vi "setUp.vi"(8 "error in (no error)":errorcluster, 11 "reference in":refnum<class "Read Value Tests.lvclass">) -> (0 "error out":errorcluster, 3 "reference out":refnum<class "Read Value Tests.lvclass">)   [LabVIEW 2020, in "Memory Manager Tests.lvlib" / "Read Value Tests.lvclass"]
doc: "setUp runs prior to the test method during test execution. Use this method to initialize any object data required by your tests."
uses:
  Read Value Tests.lvclass
  C:/Program Files (x86)/National Instruments/LabVIEW 2020/vi.lib/addons/_JKI Toolkits/VI Tester/TestCase.llb/TestCase.lvclass
  Read Value Tests.lvclass/Read Value Tests.ctl
  Source/Classes/Pointer/Write 1D U8.vi
  <vilib>/addons/_JKI Toolkits/VI Tester/TestCase.llb/TestCase.lvclass
  Source/Classes/Pointer/Pointer.lvclass
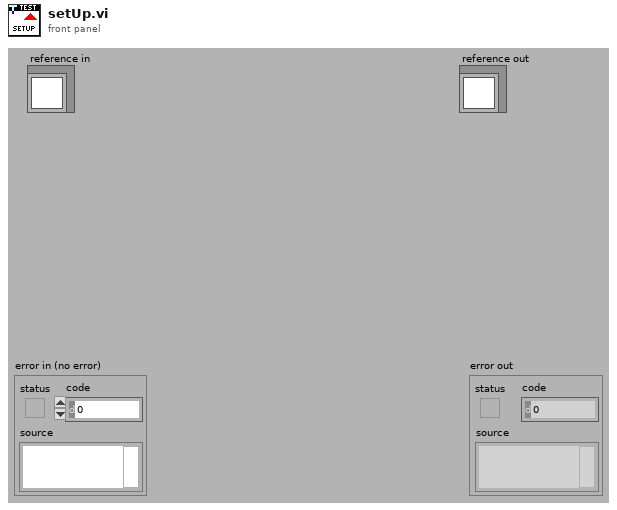
[diagram p1: front panel]
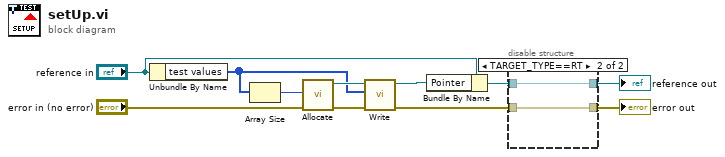
[diagram p0: block diagram]
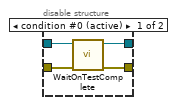
[diagram p2: hidden frame]
diagram:
  n1 = Unbundle By Name("reference in") -> ("test values"=w1:u8[])
  n2 = Array Size(array=w1) -> (size(s)=w5:i32)
  n3 = call "Allocate.vi"("error in (no error)"="error in (no error)", "size"=w5) -> ("error out"=w3:errorcluster, "Pointer out"=w8:refnum<class "Pointer.lvclass">)  [unwired: 8 in]
  n4 = call-poly "Write.vi"("error in (no error)"=w3, "buffer in"=w1, "Pointer in"=w8) -> ("error out"=w2:errorcluster, "Pointer out"=w6:refnum<class "Pointer.lvclass">)  [unwired: 5 in, 2 out]
  n5 = Bundle By Name(cluster="reference in", "Pointer"=w6) -> (w9:refnum<class "Read Value Tests.lvclass">)
  n6 = disable-structure shown="TARGET_TYPE==RT" {
    disable-tunnel: w2 -> [w15 w16]
    disable-tunnel: [w14 w16] -> w11
    disable-tunnel: [w13 w17] -> w10
    disable-tunnel: w9 -> [w12 w17]
    frame condition #0 (active) {
      n7 = call <vilib>:"WaitOnTestComplete.vi"("error in (no error)"=w15, "TestCase in"=w12) -> ("error out"=w14:errorcluster, "TestCase out"=w13:refnum<class "Read Value Tests.lvclass">)  [unwired: 8 in]
    }
    frame condition #1 {
    }
  }
  "error out" <- w11
  "reference out" <- w10
